vi "G-CLI Sink.vi"(8 "error in (no error)":errorcluster, 11 "CLI Connection":refnum<class "CLI.lvclass">) -> (0 "error out":errorcluster, 3 "G-CLI Sink out":refnum<class "G-CLI Sink.lvclass">)   [LabVIEW 2020, in "LV Logging.lvlib" / "G-CLI Sink.lvclass"]
uses:
  G-CLI Sink.lvclass
  G-CLI Sink.lvclass/G-CLI Sink.ctl
  <vilib>/Wiresmith Technology/G CLI/CLI Class/CLI.lvclass
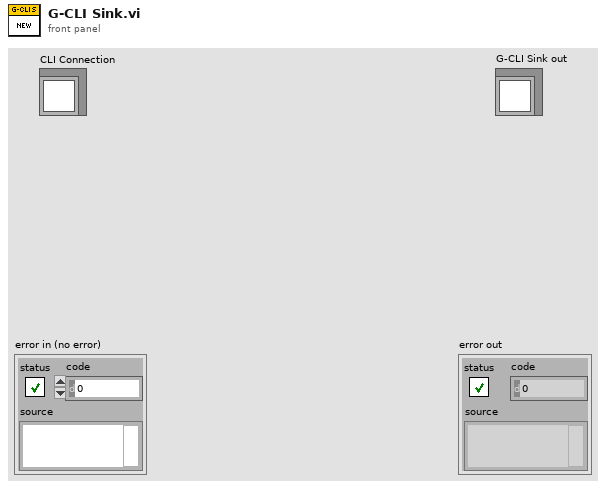
[diagram p1: front panel]
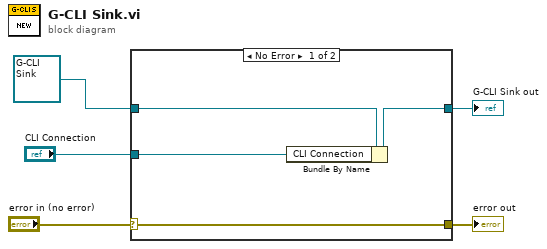
[diagram p0: block diagram]
diagram:
  n1 = case shown="No Error" "error in (no error)" {
    selector: "error in (no error)" -> [w9 w11]
    tunnel: [w9 w11] -> w4
    tunnel: [w7 w10] -> w2
    tunnel: refnum<class "G-CLI Sink.lvclass"> refnum ("G-CLI Sink in") -> [w8 w10]
    tunnel: "CLI Connection" -> [w6 _]
    frame No Error {
      n2 = Bundle By Name(cluster=w8, "CLI Connection"=w6) -> (w7:refnum<class "G-CLI Sink.lvclass">)
    }
    frame Error {
    }
  }
  "error out" <- w4
  "G-CLI Sink out" <- w2
